vi "GTLog.vi"(8 "error in (no error)":errorcluster, 11 "Numeric":i16) -> (0 "error out":errorcluster)   [LabVIEW 2020]
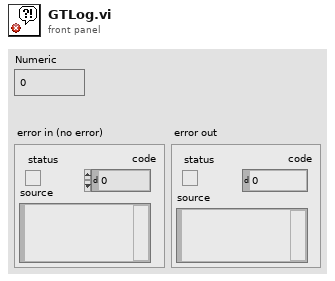
[diagram p1: front panel]
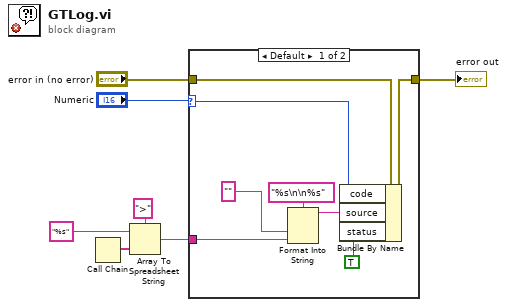
[diagram p0: block diagram]
diagram:
  n1 = Call Chain() -> (call chain=w5:string[])
  n2 = Array To Spreadsheet String(delimiter (Tab)=">", array=w5, 3:"%s" ("format string")) -> (spreadsheet string=w2:string)
  n3 = case shown="Default" "Numeric" {
    selector: "Numeric" -> [w11 _]
    tunnel: [w15 w16] -> w1
    tunnel: "error in (no error)" -> [w10 w16]
    tunnel: w2 -> [w8 _]
    frame Default {
      n4 = Format Into String(format string="%s\n\n%s", "" ("input 1"), w8) -> (resulting string=w12:string)  [unwired: 2 in, 1 out]
      n5 = Bundle By Name(cluster=w10, "code"=w11, "source"=w12, "status"=TRUE) -> (w15:errorcluster)
    }
    frame 0 {
    }
  }
  "error out" <- w1
